vi "PS VI ref.vi"(3 "error in (no error)":errorcluster) -> (0 "error out":errorcluster, 1 "vi reference":refnum<vi>)   [LabVIEW 2019]
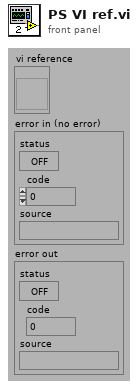
[diagram p1: front panel]
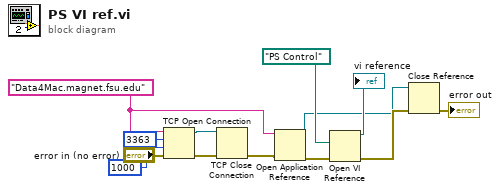
[diagram p0: block diagram]
diagram:
  w8 = "Data4Mac.magnet.fsu.edu" ("address")
  n1 = TCP Open Connection(address=w8, remote port or service name=u16 3363 ("remote port"), timeout ms (60000)=1000, error in (no error)="error in (no error)") -> (connection ID=w10:refnum<k5>, error out=w11:errorcluster)  [unwired: 1 in]
  n2 = TCP Close Connection(connection ID=w10, error in (no error)=w11) -> (error out=w9:errorcluster)  [unwired: 1 in, 1 out]
  n3 = Open Application Reference(8:w9, 11:w8) -> (0:w7:errorcluster, 3:w3:refnum<vi>)  [unwired: 2 in]
  n4 = Open VI Reference(vi path=path "PS Control", error in (no error)=w7) -> (vi reference=→"vi reference":refnum<vi>, error out=w5:errorcluster)  [unwired: 4 in]
  n5 = Close Reference(reference=w3, error in (no error)=w5) -> (error out=→"error out":errorcluster)
